vi "iSpy_server.vi"() -> ()   [LabVIEW 2018]
uses:
  Anemometry/Anemometry Sub Vis/Globals/Constants_global.vi
panel:
  out "Last Check Directories":timestamp
  in  "Video Log Interval (s)":dbl=60.0
  in  "Picture Copy Interval (s)":dbl=3.0
  out "Last Copied Pictures":timestamp
  out "Last Logged Video":timestamp
  out "Video from Here":path[](array[path])=[path "\\\\EnFlo-Data\\Public/CamServer/.AppleDouble/grabs"]
  out "error out":errorcluster
  in  "stop":bool
  out "Pictures from Here":path[](array[path])=[path "\\\\EnFlo-Data\\Public/CamServer/.AppleDouble/grabs"]
  in  "Scratch file directory":path=path "C:/CamServer/video"
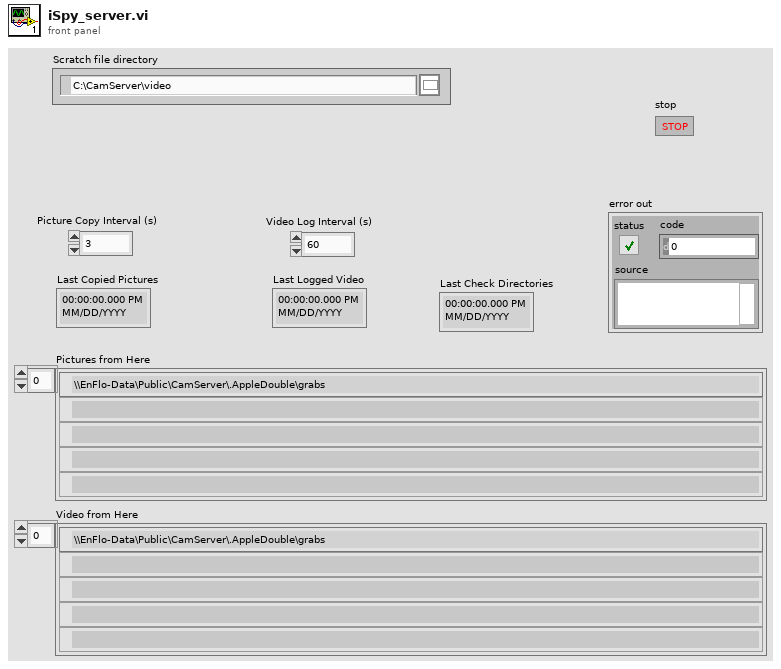
[diagram p1: front panel]
types:
  T1 = typedef "LVDateTimeRec.ctl" = cluster{"fractional second":dbl, "second":i32, "minute":i32, "hour":i32, "day of month":i32, "month":i32, "year":i32, "day of week":i32, "day of year":i32, "DST":i32}
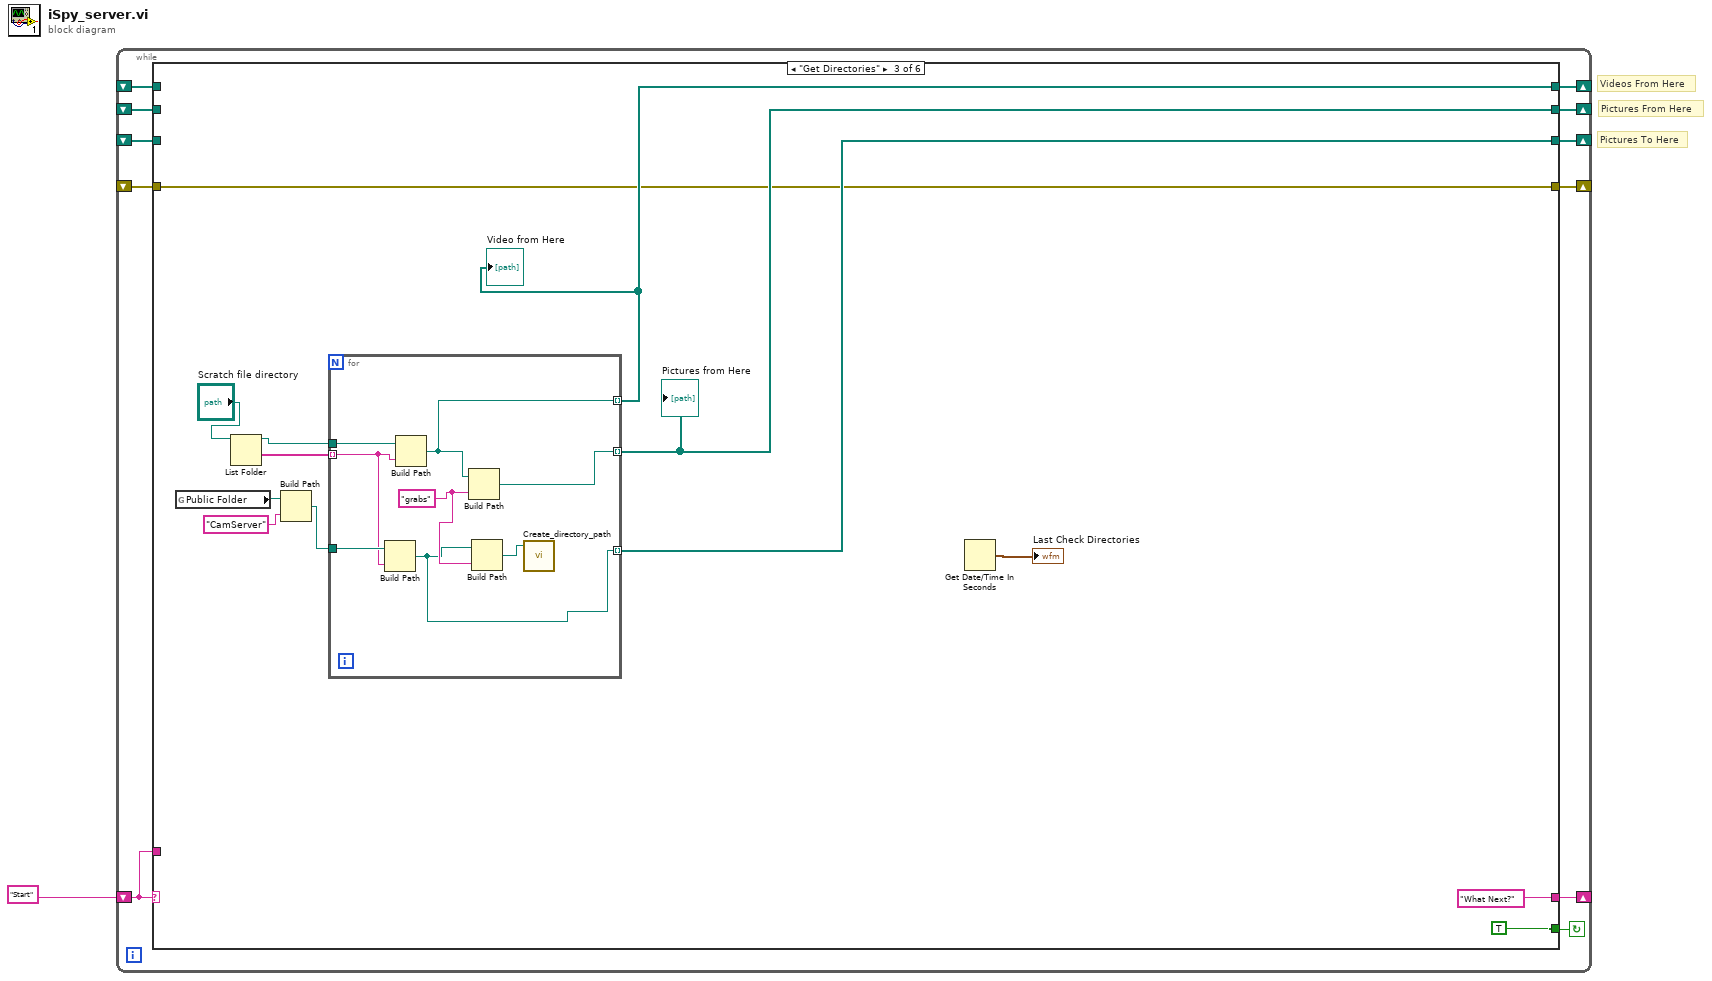
[diagram p0: block diagram]
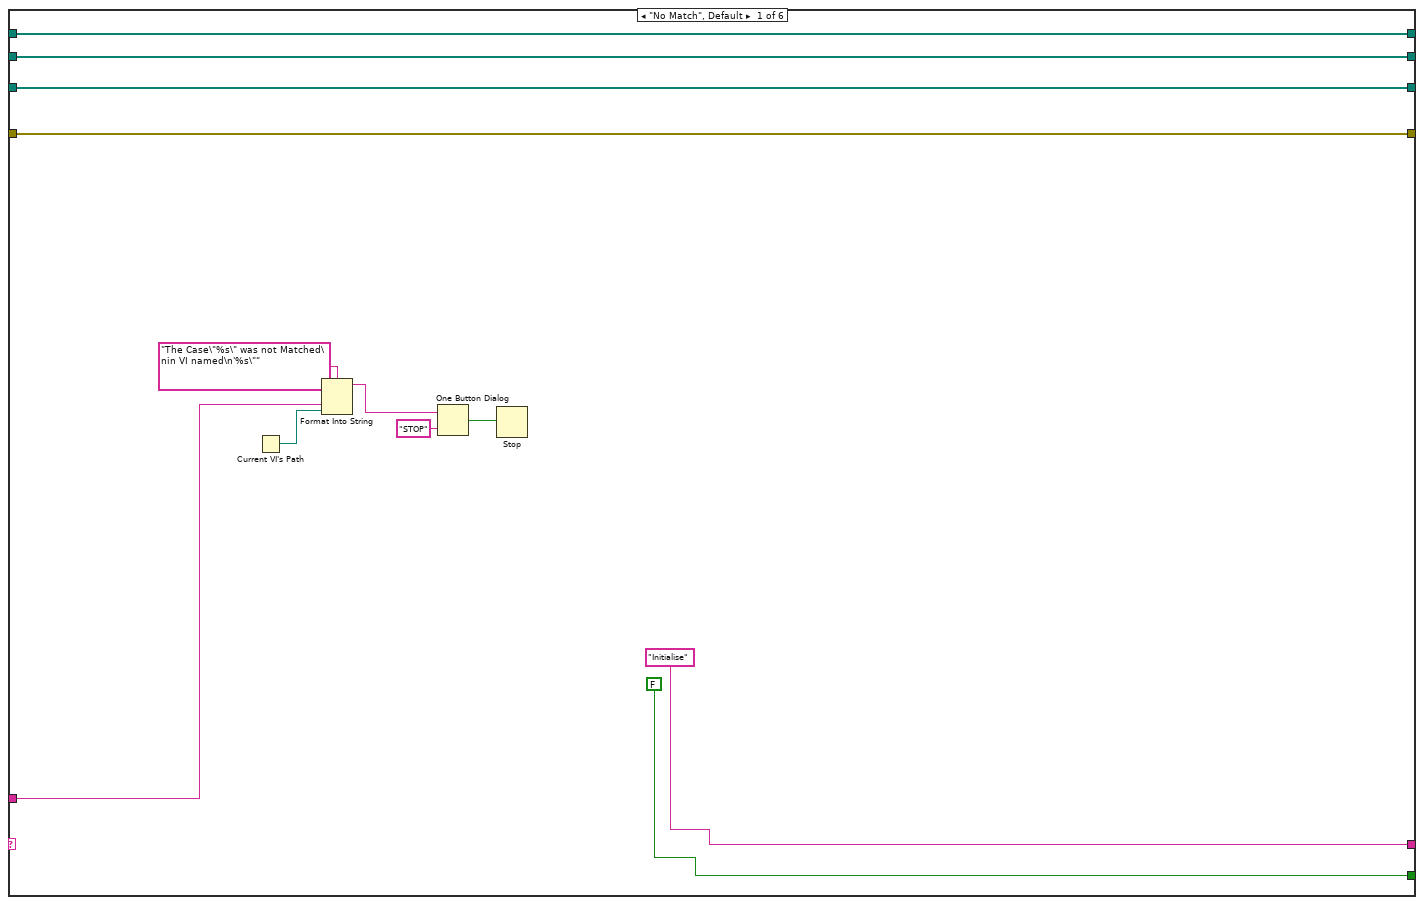
[diagram p2: hidden frame]
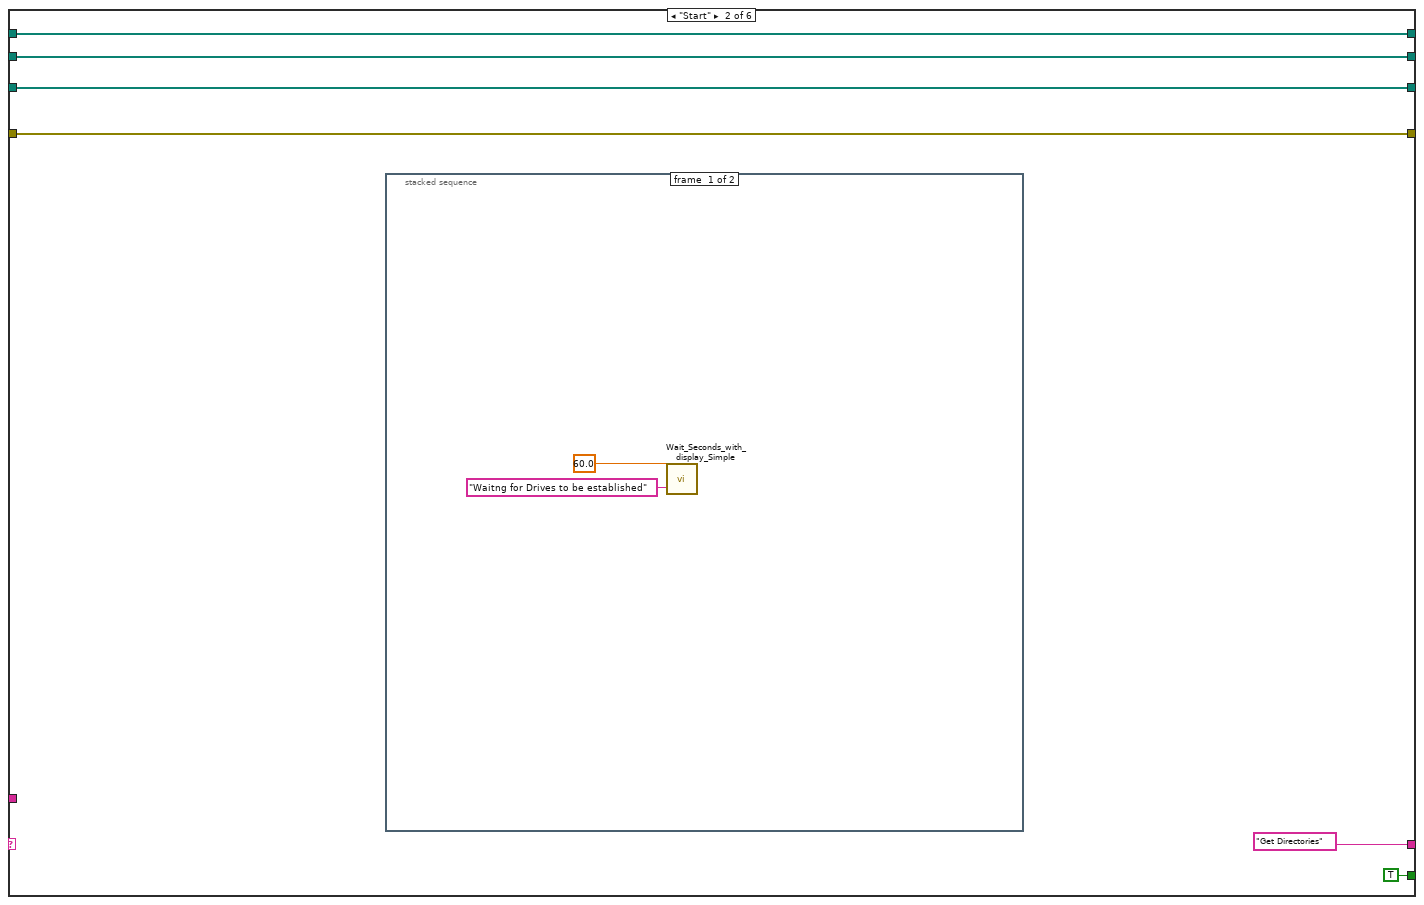
[diagram p3: hidden frame]
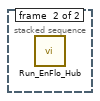
[diagram p4: hidden frame]
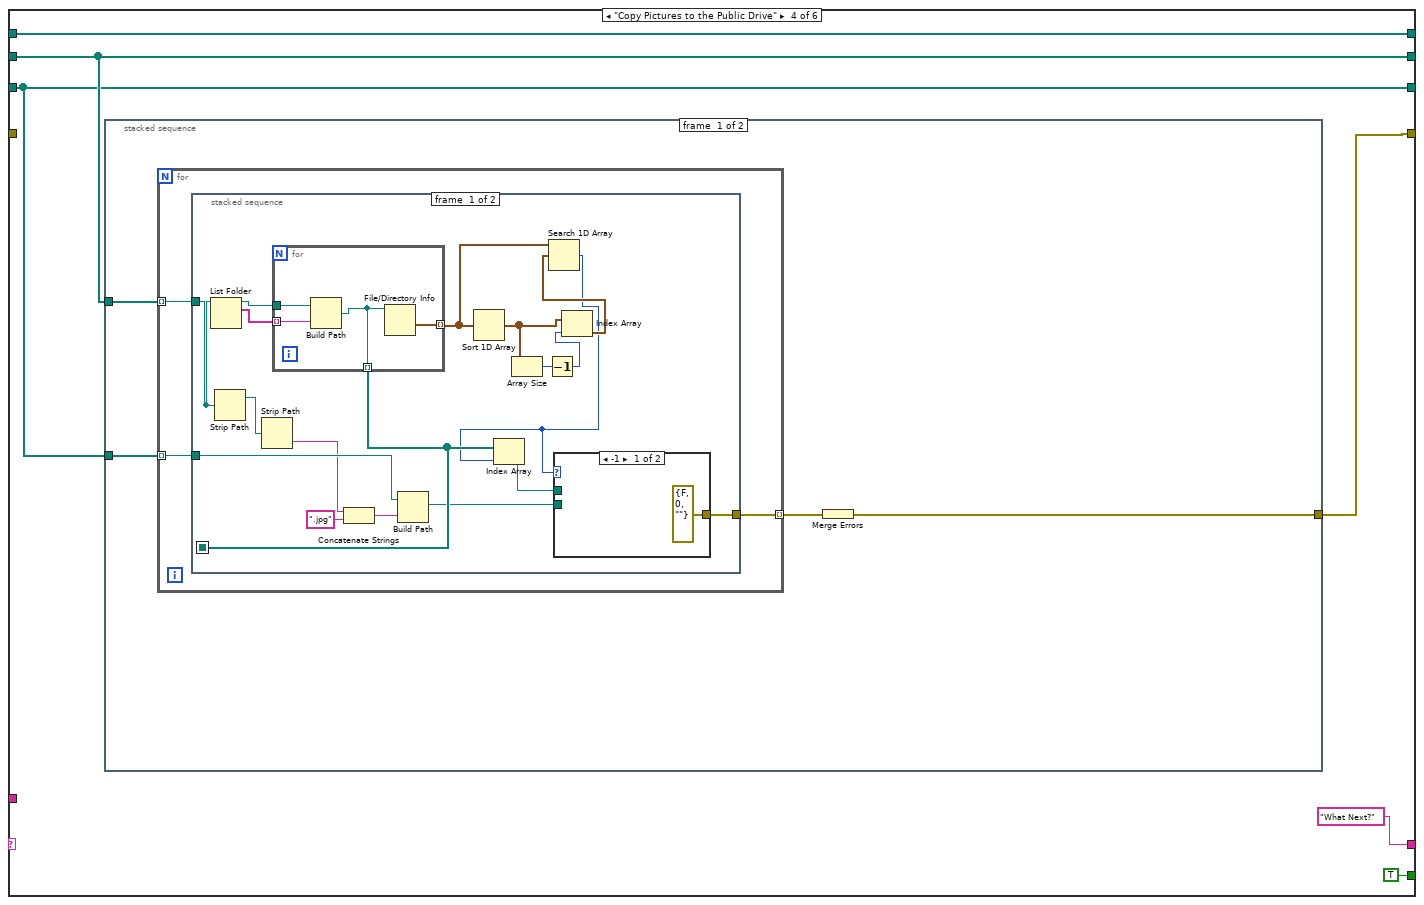
[diagram p5: hidden frame]
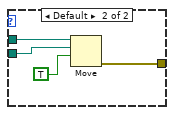
[diagram p6: hidden frame]
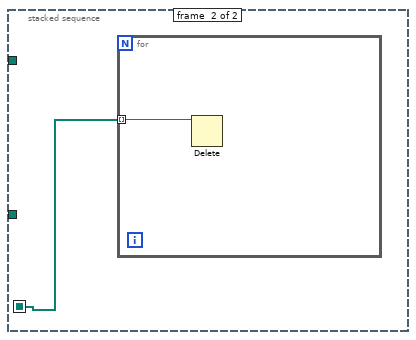
[diagram p7: hidden frame]
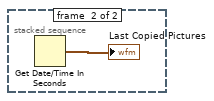
[diagram p8: hidden frame]
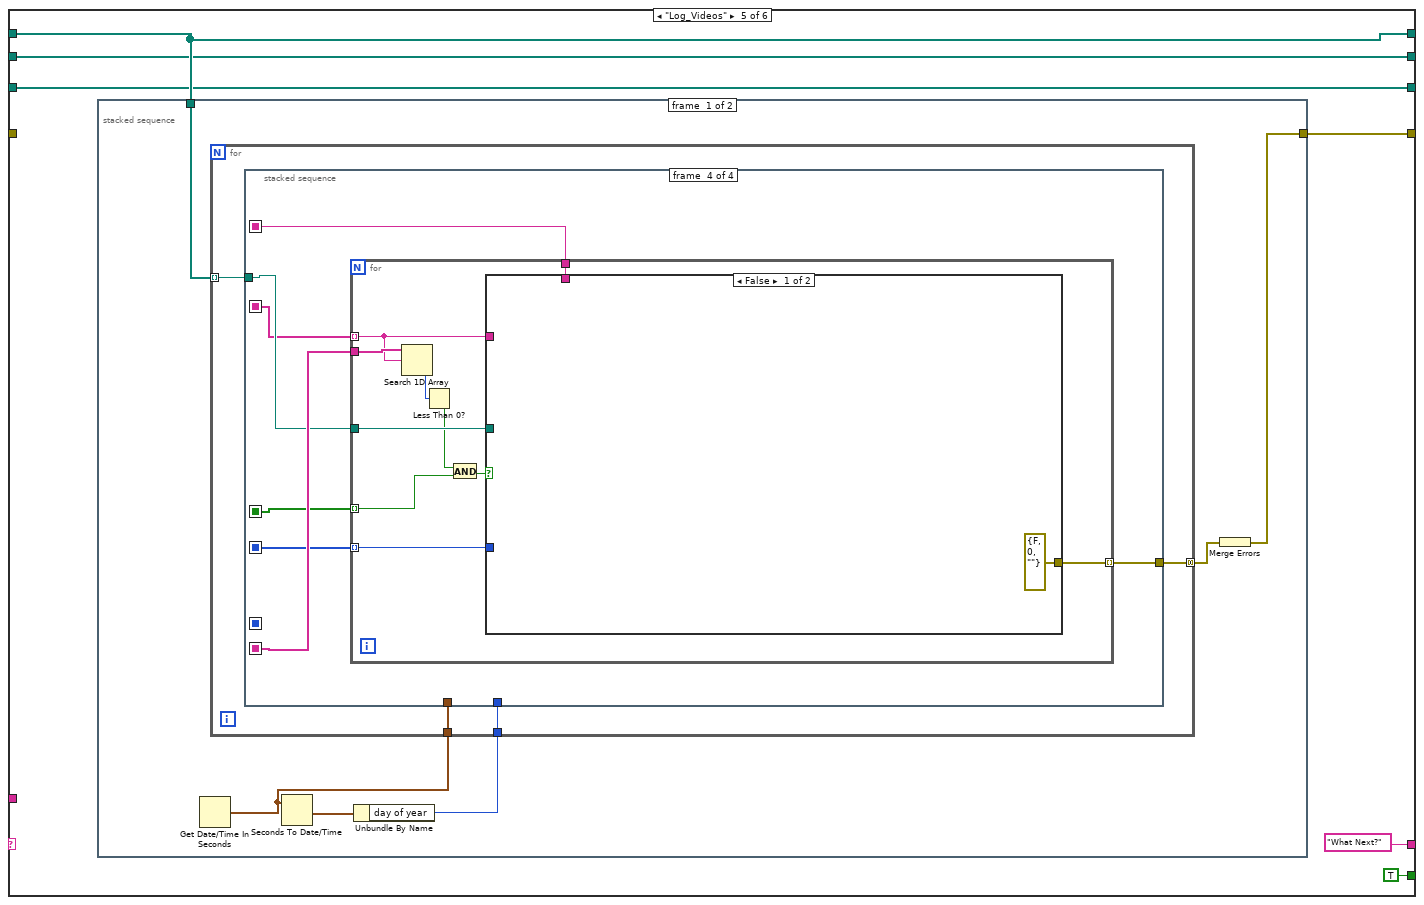
[diagram p9: hidden frame]
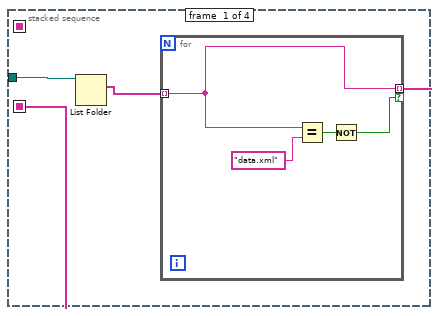
[diagram p10: hidden frame]
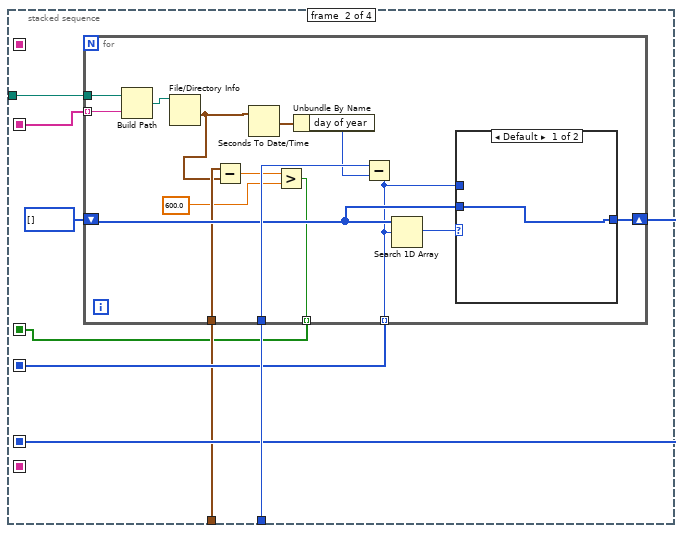
[diagram p11: hidden frame]
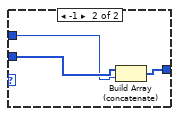
[diagram p12: hidden frame]
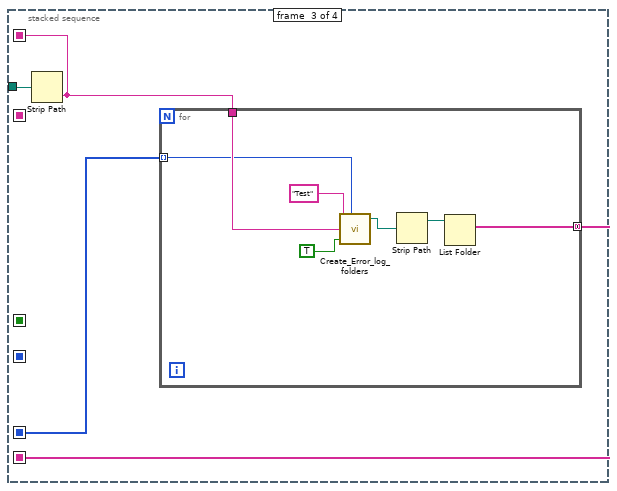
[diagram p13: hidden frame]
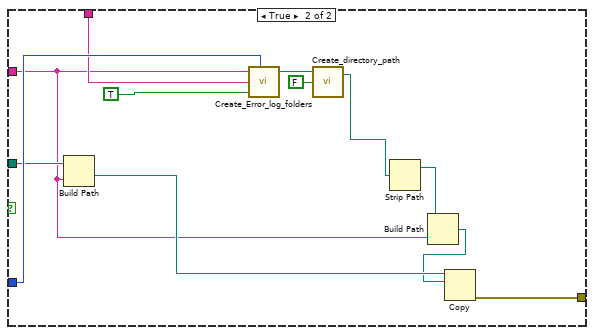
[diagram p14: hidden frame]
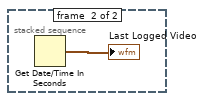
[diagram p15: hidden frame]
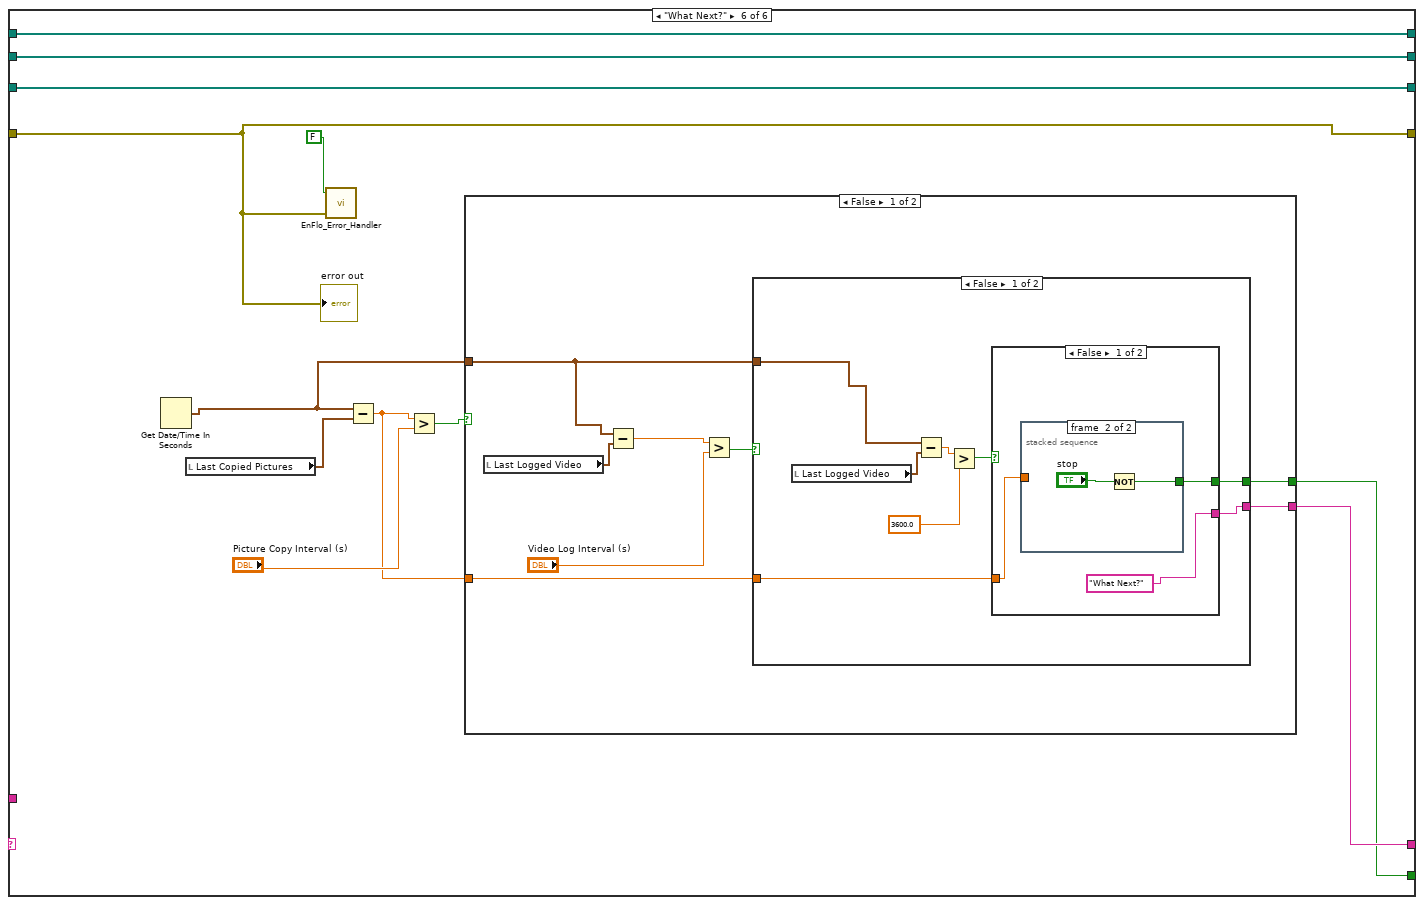
[diagram p16: hidden frame]
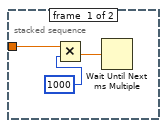
[diagram p17: hidden frame]
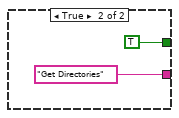
[diagram p18: hidden frame]
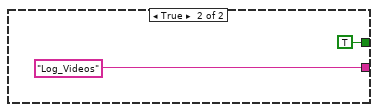
[diagram p19: hidden frame]
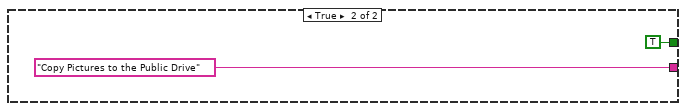
[diagram p20: hidden frame]
diagram:
  # "Videos From Here"
  # "Pictures To Here"
  # "Pictures From Here"
  n1 = while {
    shift-left: "Start" -> [w10]
    shift-right: [w11] -> _
    shift-right: [w9] -> _
    shift-left: _ -> [w8]
    shift-right: [w7] -> _
    shift-left: _ -> [w6]
    shift-right: [w5] -> _
    shift-left: _ -> [w4]
    shift-right: [w3] -> _
    shift-left: _ -> [w2]
    stop <- w12 continue-if-true
    n2 = case shown="\"Get Directories\"" w10 {
      tunnel: [FALSE TRUE ("stop") TRUE TRUE TRUE ("stop") w191] -> w12
      tunnel: ["Initialise" "Get Directories" "What Next?" "What Next?" "What Next?" w195] -> w11
      tunnel: w10 -> [w19 _ _ _ _ _]
      tunnel: [w16 w30 w41 w59 w101 w199] -> w9
      tunnel: w8 -> [w16 w30 _ w59 w101 w199]
      tunnel: [w15 w29 w40 w58 w100 w198] -> w7
      tunnel: w6 -> [w15 w29 _ w58 w100 w198]
      tunnel: [w14 w28 w38 w57 w102 w200] -> w5
      tunnel: w4 -> [w14 w28 _ w57 w102 w200]
      tunnel: [w13 w27 w36 w54 w97 w189] -> w3
      tunnel: w2 -> [w13 w27 w36 _ _ w189]
      frame "No Match", Default {
        n3 = Current VI's Path() -> (path=w18:path)
        n4 = Format Into String(format string="The Case\"%s\" was not Matched\nin VI named\n'%s\"" ("Format String"), w19, w18) -> (resulting string=w22:string)  [unwired: 2 in, 1 out]
        n5 = One Button Dialog(message=w22, button name ("OK")="STOP") -> (true=w20:bool)
        n6 = Stop(stop? (T)=w20) -> ()
      }
      frame "Start" {
        n7 = stacked-sequence {
          frame #0 {
            n8 = call "Wait_Seconds_with_display_Simple.vi"("Message"="Waitng for Drives to be established", "Seconds to wait"=60.0) -> ()  [unwired: 1 in, 1 out]
          }
          frame #1 {
            n9 = call "Run_EnFlo_Hub.vi"() -> ()  [unwired: 7 in, 1 out]
          }
        }
      }
      frame "Get Directories" {
        n10 = global read "Constants_global.vi" "Public Folder"() -> (w35:path)
        n11 = List Folder(path="Scratch file directory") -> (path out=w43:path, folder names=w42:string[])  [unwired: 3 in, 2 out]
        n12 = Build Path(base path=w35, name or relative path="CamServer") -> (appended path=w33:path)
        n13 = for {
          tunnel: w43 -> [w53]
          tunnel: w42 -> [w50] mode=indexing
          tunnel: [w52] -> w41 mode=indexing
          tunnel: w33 -> [w51]
          tunnel: [w47] -> w40 mode=indexing
          tunnel: [w46] -> w38 mode=indexing
          w49 = "grabs" ("name or relative path")
          n14 = Build Path(base path=w51, name or relative path=w50) -> (appended path=w47:path)
          n15 = Build Path(base path=w53, name or relative path=w50) -> (appended path=w46:path)
          n16 = Build Path(base path=w46, name or relative path=w49) -> (appended path=w52:path)
          n17 = Build Path(base path=w47, name or relative path=w49) -> (appended path=w48:path)
          n18 = call "Create_directory_path.vi"("Path name"=w48) -> ()  [unwired: 2 in, 2 out]
        }
        "Pictures from Here" <- w41
        "Video from Here" <- w38
        n19 = Get Date/Time In Seconds() -> (seconds since 1Jan1904=→"Last Check Directories":timestamp)
      }
      frame "Copy Pictures to the Public Drive" {
        n20 = stacked-sequence {
          tunnel: w59 -> [w63 _]
          tunnel: w58 -> [w62 _]
          tunnel: [w61 _] -> w54
          frame #0 {
            n21 = for {
              tunnel: w63 -> [w66] mode=indexing
              tunnel: w62 -> [w65] mode=indexing
              tunnel: [w64] -> w60 mode=indexing
              n22 = stacked-sequence {
                seq-local: [w72 _] -> [_ w94]
                tunnel: w66 -> [w76 _]
                tunnel: w65 -> [w75 _]
                tunnel: [w67 _] -> w64
                frame #0 {
                  n23 = List Folder(path=w76) -> (path out=w84:path, filenames=w83:string[])  [unwired: 3 in, 2 out]
                  n24 = Strip Path(path=w76) -> (stripped path=w71:path)  [unwired: 1 out]
                  n25 = Strip Path(path=w71) -> (name=w70:string)  [unwired: 1 out]
                  n26 = for {
                    tunnel: w84 -> [w93]
                    tunnel: w83 -> [w92] mode=indexing
                    tunnel: [w91] -> w82 mode=indexing
                    tunnel: [w90] -> w72 mode=indexing
                    n27 = Build Path(base path=w93, name or relative path=w92) -> (appended path=w90:path)
                    n28 = File/Directory Info(path=w90) -> (last mod=w91:timestamp)  [unwired: 1 in, 6 out]
                  }
                  n29 = Concatenate Strings(w70, ".jpg" ("string")) -> (w74:string)
                  n30 = Build Path(base path=w75, name or relative path=w74) -> (appended path=w69:path)
                  n31 = Sort 1D Array(array=w82) -> (sorted array=w79:timestamp[])
                  n32 = Array Size(array=w79) -> (size(s)=w81:i32)
                  n33 = Decrement(x=w81) -> (x-1=w80:i32)
                  n34 = Index Array(array=w79, index=w80) -> (element=w78:timestamp)
                  n35 = Search 1D Array(1D array=w82, element=w78) -> (index of element=w68:i32)  [unwired: 1 in]
                  n36 = Index Array(array=w72, index=w68) -> (element=w77:path)
                  n37 = case shown="-1" w68 {
                    tunnel: w77 -> [_ w89]
                    tunnel: w69 -> [_ w88]
                    tunnel: [errorcluster {"status"=FALSE, "code"=0, "source"=""} ("error out") w86] -> w67
                    frame -1 {
                    }
                    frame Default {
                      n38 = Move(source path=w89, 9:TRUE ("overwrite (F)"), 10:w88) -> (error out=w86:errorcluster)  [unwired: 2 in, 2 out]
                    }
                  }
                }
                frame #1 {
                  n39 = for {
                    tunnel: w94 -> [w95] mode=indexing
                    n40 = Delete(path (use dialog)=w95) -> ()  [unwired: 4 in, 3 out]
                  }
                }
              }
            }
            n41 = Merge Errors(w60) -> (w61:errorcluster)
          }
          frame #1 {
            n42 = Get Date/Time In Seconds() -> (seconds since 1Jan1904=→"Last Copied Pictures":timestamp)
          }
        }
      }
      frame "Log_Videos" {
        n43 = stacked-sequence {
          tunnel: w102 -> [w108 _]
          tunnel: [w103 _] -> w97
          frame #0 {
            n44 = Get Date/Time In Seconds() -> (seconds since 1Jan1904=w106:timestamp)
            n45 = Seconds To Date/Time(time stamp (now)=w106) -> (date time rec=w107:T1)  [unwired: 1 in]
            n46 = Unbundle By Name(w107) -> ("day of year"=w105:i32)
            n47 = for {
              tunnel: w108 -> [w112] mode=indexing
              tunnel: w105 -> [w111]
              tunnel: w106 -> [w110]
              tunnel: [w109] -> w104 mode=concatenating
              n48 = stacked-sequence {
                seq-local: [_ w125 _ _] -> [_ _ w149 _]
                seq-local: [_ _ w148 _] -> [_ _ _ w164]
                seq-local: [_ w124 _ _] -> [_ _ _ w163]
                seq-local: [_ _ w147 _] -> [_ _ _ w162]
                seq-local: [w113 _ _ _] -> [_ w123 _ w160]
                seq-local: [_ w120 _ _] -> [_ _ _ w159]
                tunnel: w112 -> [w115 w122 w150 w161]
                tunnel: w111 -> [_ w127 _ _]
                tunnel: w110 -> [_ w121 _ _]
                tunnel: [_ _ _ w158] -> w109
                frame #0 {
                  n49 = List Folder(path=w115) -> (filenames=w114:string[])  [unwired: 3 in, 3 out]
                  n50 = for {
                    tunnel: w114 -> [w118] mode=indexing
                    tunnel: [w118] -> w113 mode=indexing if=w116
                    n51 = Equal?(x=w118, y="data.xml") -> (x = y?=w117:bool)
                    n52 = Not(x=w117) -> (.not. x?=w116:bool)
                  }
                }
                frame #1 {
                  n53 = for {
                    tunnel: w122 -> [w142]
                    tunnel: w123 -> [w141] mode=indexing
                    tunnel: w127 -> [w138]
                    shift-right: [w135] -> w125
                    shift-left: i32[] [] -> [w134]
                    tunnel: [w133] -> w124 mode=indexing
                    tunnel: w121 -> [w132]
                    tunnel: [w128] -> w120 mode=indexing
                    n54 = Build Path(base path=w142, name or relative path=w141) -> (appended path=w140:path)
                    n55 = File/Directory Info(path=w140) -> (last mod=w131:timestamp)  [unwired: 1 in, 6 out]
                    n56 = Subtract(x=w132, y=w131) -> (x-y=w130:dbl)
                    n57 = Seconds To Date/Time(time stamp (now)=w131) -> (date time rec=w139:T1)  [unwired: 1 in]
                    n58 = Greater?(x=w130, y=600.0) -> (0:w128:bool)
                    n59 = Unbundle By Name(w139) -> ("day of year"=w137:i32)
                    n60 = Subtract(x=w138, y=w137) -> (x-y=w133:i32)
                    n61 = Search 1D Array(1D array=w134, element=w133) -> (index of element=w136:i32)  [unwired: 1 in]
                    n62 = case shown="Default" w136 {
                      tunnel: [w143 w146] -> w135
                      tunnel: w133 -> [_ w144]
                      tunnel: w134 -> [w143 w145]
                      frame Default {
                      }
                      frame -1 {
                        n63 = Build Array (concatenate)(w145, w144) -> (w146:i32[])
                      }
                    }
                  }
                }
                frame #2 {
                  n64 = Strip Path(path=w150) -> (name=w147:string)  [unwired: 1 out]
                  n65 = for {
                    tunnel: w147 -> [w155]
                    tunnel: w149 -> [w154] mode=indexing
                    tunnel: [w153] -> w148 mode=concatenating
                    n66 = call "Create_Error_log_folders.vi"("Log Filename"="Test", "Days ago"=w154, "Log Folder"=w155, "Per Day Log File?"=TRUE) -> ("Local Log File"=w152:path)  [unwired: 2 in, 1 out]
                    n67 = Strip Path(path=w152) -> (stripped path=w151:path)  [unwired: 1 out]
                    n68 = List Folder(path=w151) -> (filenames=w153:string[])  [unwired: 3 in, 3 out]
                  }
                }
                frame #3 {
                  n69 = for {
                    tunnel: w164 -> [w174]
                    tunnel: w160 -> [w171] mode=indexing
                    tunnel: w163 -> [w173] mode=indexing
                    tunnel: w162 -> [w172]
                    tunnel: w161 -> [w170]
                    tunnel: w159 -> [w167] mode=indexing
                    tunnel: [w165] -> w158 mode=indexing
                    n70 = Search 1D Array(1D array=w174, element=w171) -> (index of element=w169:i32)  [unwired: 1 in]
                    n71 = Less Than 0?(x=w169) -> (x < 0?=w168:bool)
                    n72 = And(x=w168, y=w167) -> (x .and. y?=w166:bool)
                    n73 = case shown="False" w166 {
                      tunnel: w173 -> [_ w186]
                      tunnel: w172 -> [_ w185]
                      tunnel: w171 -> [_ w178]
                      tunnel: w170 -> [_ w184]
                      tunnel: [errorcluster {"status"=FALSE, "code"=0, "source"=""} ("error out") w176] -> w165
                      frame False {
                      }
                      frame True {
                        n74 = Build Path(base path=w184, name or relative path=w178) -> (appended path=w183:path)
                        n75 = call "Create_Error_log_folders.vi"("Log Filename"=w178, "Days ago"=w186, "Log Folder"=w185, "Per Day Log File?"=TRUE) -> ("Local Log File"=w182:path)  [unwired: 2 in, 1 out]
                        n76 = call "Create_directory_path.vi"("Dialog Box"=FALSE, "Path name"=w182) -> ("Path name Out"=w180:path)  [unwired: 1 in, 1 out]
                        n77 = Strip Path(path=w180) -> (stripped path=w179:path)  [unwired: 1 out]
                        n78 = Build Path(base path=w179, name or relative path=w178) -> (appended path=w177:path)
                        n79 = Copy(10:w177, 11:w183) -> (0:w176:errorcluster)  [unwired: 3 in, 2 out]
                      }
                    }
                  }
                }
              }
            }
            n80 = Merge Errors(w104) -> (w103:errorcluster)
          }
          frame #1 {
            n81 = Get Date/Time In Seconds() -> (seconds since 1Jan1904=→"Last Logged Video":timestamp)
          }
        }
      }
      frame "What Next?" {
        n82 = Get Date/Time In Seconds() -> (seconds since 1Jan1904=w194:timestamp)
        n83 = local read "Last Copied Pictures"() -> (w197:timestamp)
        n84 = call "EnFlo_Error_Handler.vi"("error in (no error)"=w189, "Dialog Box (T)"=FALSE) -> ()  [unwired: 1 in, 3 out]
        n85 = Subtract(x=w194, y=w197) -> (x-y=w192:dbl)
        n86 = Greater?(x=w192, y="Picture Copy Interval (s)") -> (0:w196:bool)
        n87 = case shown="False" w196 {
          tunnel: [w204 "Copy Pictures to the Public Drive"] -> w195
          tunnel: w194 -> [w203 _]
          tunnel: w192 -> [w202 _]
          tunnel: [w201 TRUE ("stop")] -> w191
          frame False {
            n88 = local read "Last Logged Video"() -> (w208:timestamp)
            n89 = Subtract(x=w203, y=w208) -> (x-y=w207:dbl)
            n90 = Greater?(x=w207, y="Video Log Interval (s)") -> (0:w205:bool)
            n91 = case shown="False" w205 {
              tunnel: [w211 "Log_Videos"] -> w204
              tunnel: w203 -> [w215 _]
              tunnel: w202 -> [w210 _]
              tunnel: [w209 TRUE ("stop")] -> w201
              frame False {
                n92 = local read "Last Logged Video"() -> (w216:timestamp)
                n93 = Subtract(x=w215, y=w216) -> (x-y=w214:dbl)
                n94 = Greater?(x=w214, y=3600.0) -> (0:w212:bool)
                n95 = case shown="False" w212 {
                  tunnel: ["What Next?" "Get Directories"] -> w211
                  tunnel: w210 -> [w219 _]
                  tunnel: [w217 TRUE] -> w209
                  frame False {
                    n96 = stacked-sequence {
                      tunnel: w219 -> [w221 _]
                      tunnel: [_ w223] -> w217
                      frame #0 {
                        n97 = Multiply(x=w221, y=u32 1000) -> (x*y=w220:dbl)
                        n98 = Wait Until Next ms Multiple(millisecond multiple=w220) -> ()  [unwired: 1 out]
                      }
                      frame #1 {
                        n99 = Not(x="stop") -> (.not. x?=w223:bool)
                      }
                    }
                  }
                  frame True {
                  }
                }
              }
              frame True {
              }
            }
          }
          frame True {
          }
        }
        "error out" <- w189
      }
    }
  }
